vi "Single Platform.vi"(8 "error in (no error)":errorcluster, 10 "Platform Name":string, 11 "PlatformManager in":refnum<class "PlatformManager.lvclass">) -> (0 "error out":errorcluster, 2 "Platform":refnum<class "Platform.lvclass">, 3 "PlatformManager out":refnum<class "PlatformManager.lvclass">)   [LabVIEW 2020, in "PicoG-Core.lvlib" / "PlatformManager.lvclass"]
uses:
  PlatformManager.lvclass
  Platform/Platform.lvclass
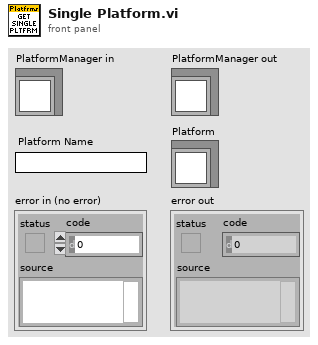
[diagram p1: front panel]
types:
  T1 = typedef "PicoG-Core.lvlib/PlatformManager.lvclass/Ref Data.ctl" = cluster{"Platforms":refnum<class "Platform.lvclass">[]}
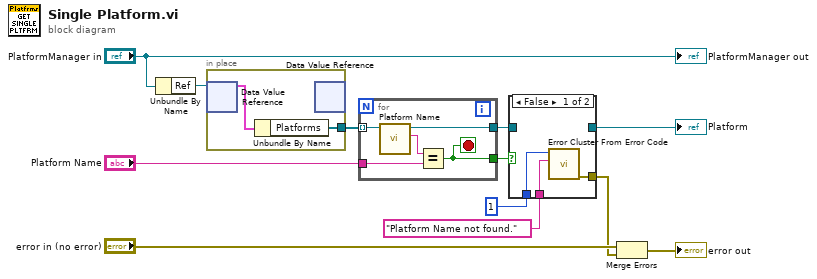
[diagram p0: block diagram]
diagram:
  n1 = Unbundle By Name("PlatformManager in") -> ("Ref"=w11:refnum<data-value>)
  n2 = in-place {
    in-place-border: [w13] -> w8
    n3 = in-place-dvr #1(w11) -> (w14:T1)  [unwired: 1 out]
    n4 = Unbundle By Name(w14) -> ("Platforms"=w13:refnum<class "Platform.lvclass">[])
    n5 = in-place-dvr #1() -> ()  [unwired: 1 in, 2 out]
  }
  n6 = for {
    tunnel: "Platform Name" -> [w18]
    tunnel: w8 -> [w19] mode=indexing
    tunnel: [w16] -> w6
    tunnel: [w15] -> w7
    stop <- w15 stop-if-true
    n7 = call-dynamic "Platform Name.vi"("DeployTarget in"=w19) -> ("Platform Name"=w17:string, "DeployTarget out"=w16:refnum<class "Platform.lvclass">)  [unwired: 8 in, 1 out]
    n8 = Equal?(x=w17, y=w18) -> (x = y?=w15:bool)
  }
  n9 = case shown="False" w7 {
    tunnel: w6 -> [_ w23]
    tunnel: [_ w23] -> w5
    tunnel: 1 -> [w22 _]
    tunnel: "Platform Name not found." -> [w21 _]
    tunnel: [w20 _] -> w1
    frame False {
      n10 = call <vilib>:"Error Cluster From Error Code.vi"("error message (\"\")"=w21, "error code (0)"=w22) -> ("error out"=w20:errorcluster)  [unwired: 7 in]
    }
    frame True {
    }
  }
  "Platform" <- w5
  n11 = Merge Errors("error in (no error)", w1) -> (→"error out":errorcluster)
  "PlatformManager out" <- "PlatformManager in"
